vi "Set Security Level.vi"(8 "error in (no error)":errorcluster, 10 "New Level":T1, 11 "Security System in":refnum<class "Security System.lvclass">) -> (0 "error out":errorcluster, 2 "Last Action Performed":string, 3 "Security System out":refnum<class "Security System.lvclass">)   [LabVIEW 2014, in "Security System.lvclass"]
uses:
  Security System.lvclass
  Security Level.ctl
  Set or Clear.ctl
  Security System.lvclass/Security System.ctl
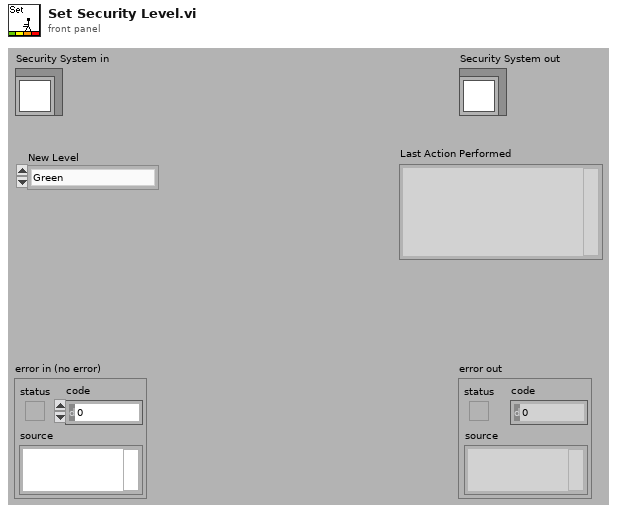
[diagram p1: front panel]
types:
  T1 = typedef "Security System.lvclass/Security Level.ctl" = enum16{"Green", "Yellow", "Orange", "Red"}
  T2 = typedef "Security System.lvclass/Set or Clear.ctl" = enum16{"Set", "Clear"}
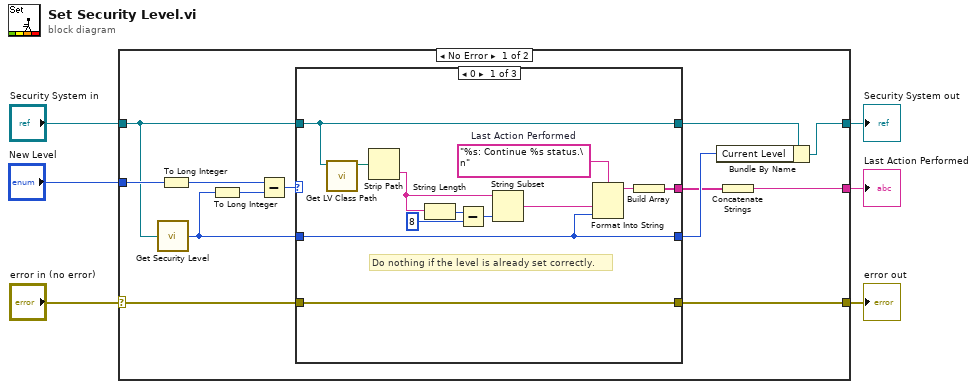
[diagram p0: block diagram]
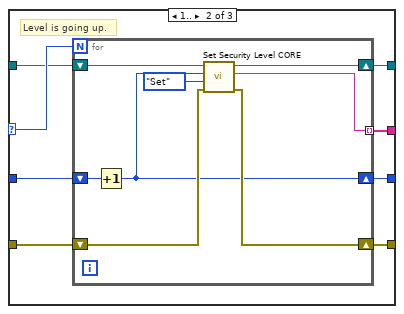
[diagram p2: hidden frame]
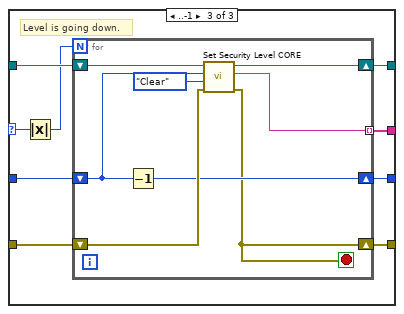
[diagram p3: hidden frame]
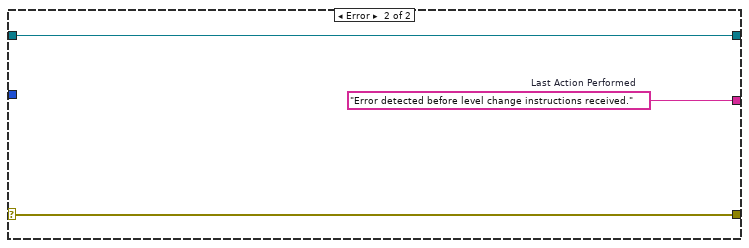
[diagram p4: hidden frame]
diagram:
  n1 = case shown="No Error" "error in (no error)" {
    selector: "error in (no error)" -> [w13 w67]
    tunnel: [w12 w67] -> w5
    tunnel: [w10 w66] -> w3
    tunnel: "Security System in" -> [w14 w66]
    tunnel: "New Level" -> [w17 _]
    tunnel: [w7 w65] -> w1
    frame No Error {
      n2 = call "Get Security Level.vi"("Security System in"=w14) -> ("Current Level"=w15:T1)
      n3 = To Long Integer(number=w17) -> (32bit integer=w16:i32)
      n4 = To Long Integer(number=w15) -> (32bit integer=w18:i32)
      n5 = Subtract(x=w16, y=w18) -> (x-y=w19:i32)
      n6 = case shown="0" w19 {
        selector: w19 -> [_ w39 w51]
        tunnel: w15 -> [w20 w38 w56]
        tunnel: w14 -> [w28 w37 w55]
        tunnel: [w28 w36 w54] -> w11
        tunnel: w13 -> [w31 w35 w53]
        tunnel: [w31 w34 w52] -> w12
        tunnel: [w20 w33 w49] -> w9
        tunnel: [w30 w32 w48] -> w8
        frame 0 {
          w25 = "%s: Continue %s status.\n"  # Last Action Performed
          # "Do nothing if the level is already set correctly."
          n7 = call <vilib>:"Get LV Class Path.vi"("object"=w28) -> ("class path"=w27:path)  [unwired: 9 in, 1 out]
          n8 = Strip Path(path=w27) -> (name=w26:string)  [unwired: 1 out]
          n9 = String Length(string=w26) -> (length=w24:i32)
          n10 = Subtract(x=w24, y=8) -> (x-y=w22:i32)
          n11 = String Subset(string=w26, length (rest)=w22) -> (substring=w21:string)  [unwired: 1 in]
          n12 = Format Into String(format string=w25, w21, w20) -> (resulting string=w29:string)  [unwired: 2 in, 1 out]
          n13 = Build Array(w29) -> (w30:string[])
        }
        frame 1.. {
          # "Level is going up."
          n14 = for {
            N: w39 -> [_]
            shift-right: [w42] -> w33
            shift-left: w38 -> [w47]
            shift-right: [w41] -> w36
            shift-left: w37 -> [w46]
            shift-right: [w44] -> w34
            shift-left: w35 -> [w45]
            tunnel: [w40] -> w32 mode=indexing
            n15 = Increment(x=w47) -> (x+1=w42:T1)
            n16 = call-dynamic "Set Security Level CORE.vi"("error in (no error)"=w45, "Set or Clear"=Set_or_Clear."Set", "New Level"=w42, "Security System in"=w46) -> ("error out"=w44:errorcluster, "Last Action Performed"=w40:string, "Security System out"=w41:refnum<class "Security System.lvclass">)  [unwired: 5 in]
          }
        }
        frame ..-1 {
          # "Level is going down."
          n17 = Absolute Value(x=w51) -> (abs(x)=w50:i32)
          n18 = for {
            N: w50 -> [_]
            shift-right: [w60] -> w49
            shift-left: w56 -> [w62]
            shift-right: [w59] -> w54
            shift-left: w55 -> [w64]
            shift-right: [w58] -> w52
            shift-left: w53 -> [w63]
            tunnel: [w57] -> w48 mode=indexing
            stop <- w58 stop-if-true
            n19 = Decrement(x=w62) -> (x-1=w60:T1)
            n20 = call-dynamic "Set Security Level CORE.vi"("error in (no error)"=w63, "Set or Clear"=Set_or_Clear."Clear", "New Level"=w62, "Security System in"=w64) -> ("error out"=w58:errorcluster, "Last Action Performed"=w57:string, "Security System out"=w59:refnum<class "Security System.lvclass">)  [unwired: 5 in]
          }
        }
      }
      n21 = Bundle By Name(cluster=w11, "Current Level"=w9) -> (w10:refnum<class "Security System.lvclass">)
      n22 = Concatenate Strings(w8) -> (w7:string)
    }
    frame Error {
      w65 = "Error detected before level change instructions received."  # Last Action Performed
    }
  }
  "error out" <- w5
  "Security System out" <- w3
  "Last Action Performed" <- w1
